vi "RenderRects.vi"(8 "No Error":errorcluster, 10 "Rects":T1[](array[typedef]), 11 "Renderer [SDL_Renderer *]":T2 format="%.0x") -> (0 "error out":errorcluster)   [LabVIEW 2026, in "SDL3.lvlib" / "Render.lvlib"]
doc: "<B>Summary</B>\nDraw some number of rectangles on the current rendering target at subpixel precision."
uses:
  Render.lvlib
  Rect/FRect--cluster.ctl
  <vilib>/Utility/error.llb/Error Cluster From Error Code.vi
  Error/Error.lvlib
  Lib/SDL3.dll
  Rect/Rect.lvlib
  SDL_Renderer--pointer.ctl
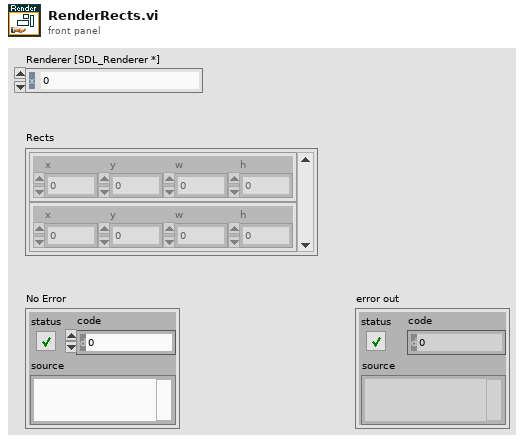
[diagram p1: front panel]
types:
  T1 = typedef "SDL3.lvlib/Rect.lvlib/FRect--cluster.ctl" = cluster{"x":sgl, "y":sgl, "w":sgl, "h":sgl}
  T2 = typedef "SDL3.lvlib/Render.lvlib/SDL_Renderer--pointer.ctl" = i64
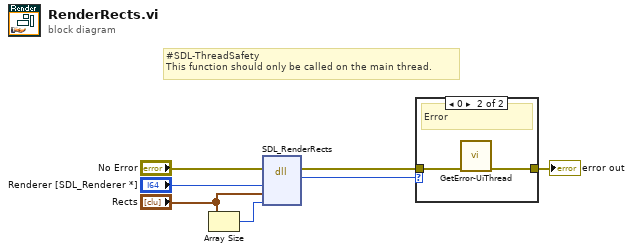
[diagram p0: block diagram]
diagram:
  # "#SDL-ThreadSafety\nThis function should only be called on the main thread."
  n1 = Array Size(array="Rects") -> (size(s)=w1:i32)
  n2 = dll-call lib="C:/Users/saukko/Dev/LV-SDL3/Sources/SDL3/Lib/SDL3.*" fn="SDL_RenderRects"(error in="No Error", "renderer"="Renderer [SDL_Renderer *]", "rects"="Rects", "count"=w1) -> (error out=w3:errorcluster, "return type"=w2:i32)  [unwired: 5 in, 1 out]
  n3 = case shown="0" w2 {
    tunnel: w3 -> [w8 w10]
    tunnel: [w8 w9] -> w6
    frame Default {
      # "Ok"
    }
    frame 0 {
      # "Error"
      n4 = call "GetError-UiThread.vi"("No Error"=w10) -> ("error out"=w9:errorcluster)  [unwired: 10 in]
    }
  }
  "error out" <- w6
